vi "auto low bar and shoot.vi"(8 "high?":bool, 9 "Distance":dbl, 10 "defenseMode":dbl, 11 "RPM setting":dbl) -> ()   [LabVIEW 2015]
uses:
  <vilib>/Rock Robotics/WPI/Solenoid/WPI_SolenoidValue.ctl
  <vilib>/Rock Robotics/WPI/CAN/TalonSRX/WPI_CANTalonSRX_APIControlMode.ctl
  <vilib>/Rock Robotics/WPI/Solenoid/WPI_SolenoidSetEnum.vi
  <vilib>/Rock Robotics/Network Tables/NT Read Number.vi
  <vilib>/Rock Robotics/Network Tables/NT Read Boolean.vi
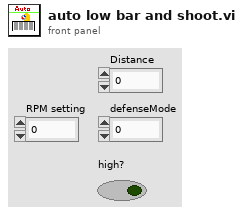
[diagram p1: front panel]
types:
  T1 = typedef "WPI_MotorControlDeviceRef.ctl" = cluster{"DeviceStatus":errorcluster, "Type":T2, "PWM":cluster{"PWM Channel":T3, "DeadBand":T4}, "CAN":cluster{"Device Number":u8, "Control Mode":T5, "Semaphore":T6, "Max Vout":dbl, "TalonSRX Control Mode":T7}, "Invert":bool}
  T2 = typedef "WPI_MotorControlType.ctl" = enum16{"PWM", "CAN", "CANTalonSRX"}
  T3 = typedef "FPGA_DIOPWMChannel.ctl" = enum8{"PWM 0", "PWM 1", "PWM 2", "PWM 3", "PWM 4", "PWM 5", "PWM 6", "PWM 7", "PWM 8", "PWM 9", "PWM MXP 0", "PWM MXP 1", "PWM MXP 2", "PWM MXP 3", "PWM MXP 4", "PWM MXP 5", "PWM MXP 6", "PWM MXP 7", "PWM MXP 8", "PWM MXP 9", "Invalid"}
  T4 = typedef "WPI_PWMDeadband.ctl" = cluster{"Name":string, "maxPositivePwm":i32, "minPositivePwm":i32, "centerPwm":i32, "maxNegativePwm":i32, "minNegativePwm":i32, "angularRange":u16}
  T5 = typedef "WPI_CANJaguar_ControlMode.ctl" = enum8{"Percent VBus", "Current", "Speed", "Position", "Voltage"}
  T6 = typedef "Semaphore RefNum" = refnum<k1>
  T7 = typedef "WPI_CANTalonSRX_APIControlMode.ctl" = enum8{"Percent VBus", "Speed", "Position", "Slave", "Unchanged / Invalid", "Voltage Compensation", "Current", "Motion Profile"}
  T8 = typedef "WPI_SolenoidDevRef.ctl" = cluster{"DevStatus":errorcluster, "Pneumatics Control Module":u8, "Forward Solenoid Channel":T9, "Reverse Solenoid Channel":T9}
  T9 = typedef "WPI_SolenoidChannel.ctl" = enum8{"Solenoid 0", "Solenoid 1", "Solenoid 2", "Solenoid 3", "Solenoid 4", "Solenoid 5", "Solenoid 6", "Solenoid 7", "Invalid"}
  T10 = typedef "WPI_GyroDevRef.ctl" = cluster{"DevStatus":errorcluster, "Analog Channel":T11, "Offset":dbl, "Gain (VoltsPerDegree/Second)":dbl, "Gyro Type":enum16{"Analog", "XRS450"}, "Handle":i32, "SPI Bus":T12, "Device Found":bool, "Sample Rate":dbl, "Calibrate On Open":bool}
  T11 = typedef "FPGA_AIChannel.ctl" = enum8{"AI 0", "AI 1", "AI 2", "AI 3", "AI MXP 0", "AI MXP 1", "AI MXP 2", "AI MXP 3", "Invalid"}
  T12 = typedef "spi_bus.ctl" = enum16{"SPI On-Board, CS0", "SPI On-Board, CS1", "SPI On-Board, CS2", "SPI On-Board, CS3", "SPI MXP", "Invalid"}
  T13 = typedef "WPI_SolenoidValue.ctl" = enum16{"Off", "On", "Forward", "Reverse"}
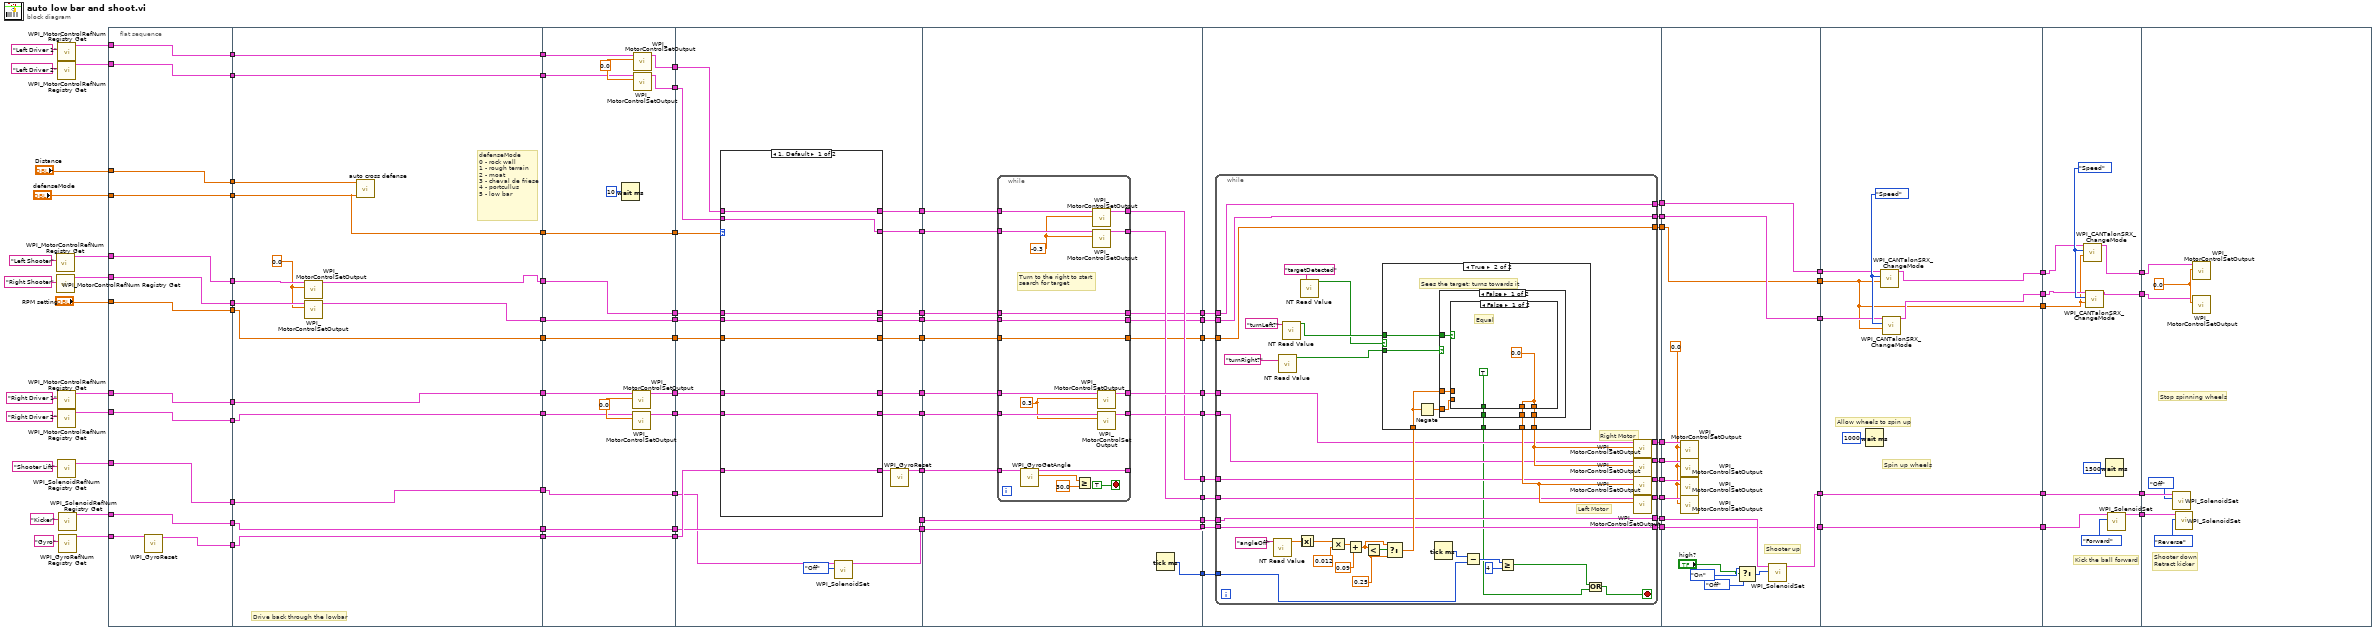
[diagram p0: block diagram]
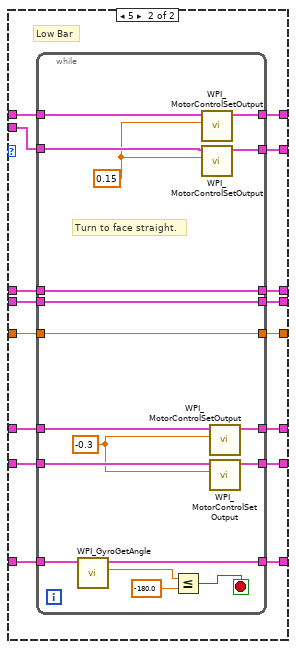
[diagram p2: hidden frame]
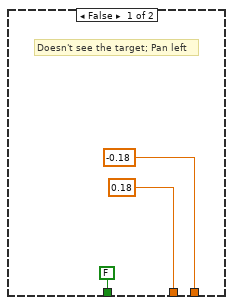
[diagram p3: hidden frame]
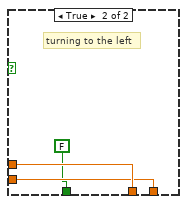
[diagram p4: hidden frame]
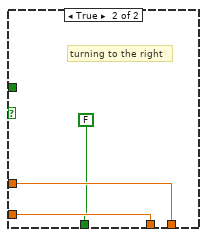
[diagram p5: hidden frame]
diagram:
  n1 = call <vilib>:"WPI_MotorControlRefNum Registry Get.vi"("refnum name"="Left Shooter") -> ("MotorControlDevRef"=w75:T1)  [unwired: 9 in, 1 out]
  n2 = call <vilib>:"WPI_MotorControlRefNum Registry Get.vi"("refnum name"="Right Shooter") -> ("MotorControlDevRef"=w72:T1)  [unwired: 9 in, 1 out]
  n3 = call <vilib>:"WPI_MotorControlRefNum Registry Get.vi"("refnum name"="Left Driver 1") -> ("MotorControlDevRef"=w98:T1)  [unwired: 9 in, 1 out]
  n4 = call <vilib>:"WPI_MotorControlRefNum Registry Get.vi"("refnum name"="Left Driver 2") -> ("MotorControlDevRef"=w97:T1)  [unwired: 9 in, 1 out]
  n5 = call <vilib>:"WPI_MotorControlRefNum Registry Get.vi"("refnum name"="Right Driver 1") -> ("MotorControlDevRef"=w96:T1)  [unwired: 9 in, 1 out]
  n6 = call <vilib>:"WPI_MotorControlRefNum Registry Get.vi"("refnum name"="Right Driver 2") -> ("MotorControlDevRef"=w95:T1)  [unwired: 9 in, 1 out]
  n7 = call <vilib>:"WPI_SolenoidRefNum Registry Get.vi"("refnum name"="Shooter Lift") -> ("SolenoidDevRef"=w90:T8)  [unwired: 9 in, 1 out]
  n8 = call <vilib>:"WPI_SolenoidRefNum Registry Get.vi"("refnum name"="Kicker") -> ("SolenoidDevRef"=w68:T8)  [unwired: 9 in, 1 out]
  n9 = call <vilib>:"WPI_GyroRefNum Registry Get.vi"("refnum name"="Gyro") -> ("GyroDevRef"=w86:T10)  [unwired: 9 in, 1 out]
  n10 = flat-sequence {
    tunnel: w95 -> [w108]
    tunnel: w96 -> [w109]
    tunnel: w97 -> [w110]
    tunnel: w98 -> [w111]
    tunnel: [w111] -> w94
    tunnel: [w110] -> w93
    tunnel: [w109] -> w92
    tunnel: [w108] -> w91
    tunnel: w90 -> [w99]
    tunnel: [w102] -> w87
    tunnel: w86 -> [w103]
    tunnel: [w107] -> w76
    tunnel: w75 -> [w107]
    tunnel: "RPM setting" -> [w106]
    tunnel: [w106] -> w73
    tunnel: w72 -> [w105]
    tunnel: [w105] -> w71
    tunnel: [w104] -> w69
    tunnel: w68 -> [w104]
    tunnel: [w99] -> w58
    tunnel: [w101] -> w57
    tunnel: "defenseMode" -> [w101]
    tunnel: "Distance" -> [w100]
    tunnel: [w100] -> w46
    tunnel: w94 -> [w126]
    tunnel: w93 -> [w125]
    tunnel: w92 -> [w122]
    tunnel: w91 -> [w121]
    tunnel: w87 -> [w119]
    tunnel: w76 -> [w116]
    tunnel: w73 -> [w124]
    tunnel: w71 -> [w115]
    tunnel: w69 -> [w118]
    tunnel: w58 -> [w120]
    tunnel: w57 -> [w117]
    tunnel: [w126] -> w55
    tunnel: [w125] -> w54
    tunnel: [w114] -> w52
    tunnel: [w113] -> w51
    tunnel: [w124] -> w49
    tunnel: w46 -> [w123]
    tunnel: [w122] -> w45
    tunnel: [w121] -> w44
    tunnel: [w120] -> w43
    tunnel: [w119] -> w41
    tunnel: [w118] -> w40
    tunnel: [w117] -> w36
    tunnel: [w142] -> w85
    tunnel: [w141] -> w84
    tunnel: [w140] -> w83
    tunnel: [w139] -> w82
    tunnel: [w128] -> w77
    tunnel: w55 -> [w137]
    tunnel: w54 -> [w136]
    tunnel: [w135] -> w53
    tunnel: w52 -> [w135]
    tunnel: w51 -> [w134]
    tunnel: [w134] -> w50
    tunnel: w49 -> [w133]
    tunnel: [w133] -> w48
    tunnel: w45 -> [w132]
    tunnel: w44 -> [w131]
    tunnel: w43 -> [w128]
    tunnel: [w130] -> w42
    tunnel: w41 -> [w130]
    tunnel: w40 -> [w129]
    tunnel: [w129] -> w39
    tunnel: [w127] -> w37
    tunnel: w36 -> [w127]
    tunnel: w85 -> [w163]
    tunnel: w84 -> [w162]
    tunnel: w83 -> [w165]
    tunnel: w82 -> [w164]
    tunnel: w77 -> [w153]
    tunnel: w53 -> [w152]
    tunnel: w50 -> [w150]
    tunnel: w48 -> [w148]
    tunnel: w42 -> [w161]
    tunnel: w39 -> [w154]
    tunnel: w37 -> [w166]
    tunnel: [w159] -> w35
    tunnel: [w158] -> w34
    tunnel: [w157] -> w33
    tunnel: [w156] -> w32
    tunnel: [w155] -> w31
    tunnel: [w154] -> w21
    tunnel: [w146] -> w19
    tunnel: [w151] -> w14
    tunnel: [w149] -> w13
    tunnel: [w147] -> w12
    tunnel: w35 -> [w226]
    tunnel: w34 -> [w225]
    tunnel: w33 -> [w224]
    tunnel: w32 -> [w223]
    tunnel: w31 -> [w222]
    tunnel: [w221] -> w30
    tunnel: [w220] -> w29
    tunnel: [w219] -> w28
    tunnel: [w218] -> w27
    tunnel: [w217] -> w22
    tunnel: w21 -> [w217]
    tunnel: w19 -> [w216]
    tunnel: [w216] -> w18
    tunnel: w14 -> [w215]
    tunnel: w13 -> [w214]
    tunnel: w12 -> [w213]
    tunnel: [w212] -> w10
    tunnel: [w211] -> w8
    tunnel: [w210] -> w6
    tunnel: [w209] -> w1
    tunnel: w30 -> [w263]
    tunnel: w29 -> [w262]
    tunnel: w28 -> [w261]
    tunnel: w27 -> [w260]
    tunnel: [w259] -> w26
    tunnel: [w258] -> w25
    tunnel: [w257] -> w24
    tunnel: [w256] -> w23
    tunnel: w22 -> [w255]
    tunnel: [w254] -> w20
    tunnel: w18 -> [w253]
    tunnel: [w252] -> w17
    tunnel: [w251] -> w11
    tunnel: w10 -> [w250]
    tunnel: [w249] -> w9
    tunnel: w8 -> [w248]
    tunnel: [w247] -> w7
    tunnel: w6 -> [w246]
    tunnel: w1 -> [w245]
    tunnel: [w336] -> w38
    tunnel: w26 -> [w335]
    tunnel: w25 -> [w334]
    tunnel: w24 -> [w333]
    tunnel: w23 -> [w332]
    tunnel: w20 -> [w329]
    tunnel: w17 -> [w330]
    tunnel: [w329] -> w15
    tunnel: w11 -> [w328]
    tunnel: w9 -> [w327]
    tunnel: w7 -> [w326]
    tunnel: [w328] -> w5
    tunnel: [w327] -> w4
    tunnel: [w326] -> w3
    tunnel: w38 -> [w348]
    tunnel: [w348] -> w66
    tunnel: [w347] -> w64
    tunnel: [w346] -> w62
    tunnel: [w344] -> w16
    tunnel: w15 -> [w344]
    tunnel: w5 -> [w343]
    tunnel: w4 -> [w342]
    tunnel: w3 -> [w341]
    tunnel: [w341] -> w2
    tunnel: [w358] -> w67
    tunnel: w66 -> [w358]
    tunnel: [w355] -> w65
    tunnel: w64 -> [w353]
    tunnel: [w354] -> w63
    tunnel: w62 -> [w352]
    tunnel: [w357] -> w61
    tunnel: w16 -> [w351]
    tunnel: w2 -> [w350]
    tunnel: w67 -> [w367]
    tunnel: w65 -> [w361]
    tunnel: w63 -> [w362]
    tunnel: w61 -> [w365]
    frame #0 {
      n11 = call <vilib>:"WPI_GyroReset.vi"("GyroDevRef"=w103) -> ("GyroDevRef"=w102:T10)  [unwired: 9 in, 1 out]
    }
    frame #1 {
      w112 = 0.0 ("Output")
      # "defenseMode\n0 - rock wall\n1 - rough terrain\n2 - moat\n3 - cheval de friese\n4 - portcullus\n5 - low bar"
      # "Drive back through the lowbar"
      n12 = call <vilib>:"WPI_MotorControlSetOutput.vi"("Output"=w112, "MotorControlDevRef"=w116) -> ("MotorControlDevRef"=w114:T1)  [unwired: 7 in, 2 out]
      n13 = call <vilib>:"WPI_MotorControlSetOutput.vi"("Output"=w112, "MotorControlDevRef"=w115) -> ("MotorControlDevRef"=w113:T1)  [unwired: 7 in, 2 out]
      n14 = call "auto cross defense.vi"("Defense type"=w117, "Distance"=w123) -> ()  [unwired: 10 in]
    }
    frame #2 {
      w143 = 0.0
      w144 = 0.0
      n15 = Wait (ms)(milliseconds to wait=u32 10) -> ()  [unwired: 1 out]
      n16 = call <vilib>:"WPI_MotorControlSetOutput.vi"("Output"=w143, "MotorControlDevRef"=w132) -> ("MotorControlDevRef"=w140:T1)  [unwired: 7 in, 2 out]
      n17 = call <vilib>:"WPI_MotorControlSetOutput.vi"("Output"=w143, "MotorControlDevRef"=w131) -> ("MotorControlDevRef"=w139:T1)  [unwired: 7 in, 2 out]
      n18 = call <vilib>:"WPI_MotorControlSetOutput.vi"("Output"=w144, "MotorControlDevRef"=w137) -> ("MotorControlDevRef"=w142:T1)  [unwired: 7 in, 2 out]
      n19 = call <vilib>:"WPI_MotorControlSetOutput.vi"("Output"=w144, "MotorControlDevRef"=w136) -> ("MotorControlDevRef"=w141:T1)  [unwired: 7 in, 2 out]
    }
    frame #3 {
      n20 = case shown="1, Default" w166 {
        tunnel: w165 -> [w171 w190]
        tunnel: w164 -> [w170 w189]
        tunnel: w163 -> [w173 w188]
        tunnel: w162 -> [w172 w187]
        tunnel: w161 -> [w174 w186]
        tunnel: [w174 w185] -> w160
        tunnel: [w171 w184] -> w158
        tunnel: [w170 w183] -> w157
        tunnel: [w173 w182] -> w156
        tunnel: [w172 w181] -> w155
        tunnel: w152 -> [w169 w180]
        tunnel: [w169 w179] -> w151
        tunnel: w150 -> [w168 w178]
        tunnel: [w168 w177] -> w149
        tunnel: [w167 w175] -> w147
        tunnel: w148 -> [w167 w176]
        frame 1, Default {
        }
        frame 5 {
          # "Low Bar"
          n21 = while {
            tunnel: w190 -> [w205]
            tunnel: w189 -> [w204]
            tunnel: w188 -> [w203]
            tunnel: w187 -> [w202]
            tunnel: w186 -> [w199]
            tunnel: [w198] -> w185
            tunnel: [w197] -> w184
            tunnel: [w196] -> w183
            tunnel: [w195] -> w182
            tunnel: [w194] -> w181
            tunnel: [w193] -> w179
            tunnel: w180 -> [w193]
            tunnel: [w192] -> w177
            tunnel: w178 -> [w192]
            tunnel: w176 -> [w191]
            tunnel: [w191] -> w175
            stop <- w208 stop-if-true
            w201 = -0.3 ("Output")
            w200 = 0.15
            # "Turn to face straight."
            n22 = call <vilib>:"WPI_GyroGetAngle.vi"("GyroDevRef"=w199) -> ("Angle"=w207:dbl, "GyroDevRef"=w198:T10)  [unwired: 6 in, 3 out]
            n23 = Less Or Equal?(x=w207, y=-180.0) -> (x <= y?=w208:bool)
            n24 = call <vilib>:"WPI_MotorControlSetOutput.vi"("Output"=w200, "MotorControlDevRef"=w203) -> ("MotorControlDevRef"=w195:T1)  [unwired: 7 in, 2 out]
            n25 = call <vilib>:"WPI_MotorControlSetOutput.vi"("Output"=w200, "MotorControlDevRef"=w202) -> ("MotorControlDevRef"=w194:T1)  [unwired: 7 in, 2 out]
            n26 = call <vilib>:"WPI_MotorControlSetOutput.vi"("Output"=w201, "MotorControlDevRef"=w205) -> ("MotorControlDevRef"=w197:T1)  [unwired: 7 in, 2 out]
            n27 = call <vilib>:"WPI_MotorControlSetOutput.vi"("Output"=w201, "MotorControlDevRef"=w204) -> ("MotorControlDevRef"=w196:T1)  [unwired: 7 in, 2 out]
          }
        }
      }
      n28 = call-poly <vilib>:"WPI_SolenoidSet.vi"("Value"=WPI_SolenoidValue."Off", "SolenoidDevRef"=w153) -> ("SolenoidDevRef"=w146:T8)  [unwired: 8 in, 1 out]
      n29 = call <vilib>:"WPI_GyroReset.vi"("GyroDevRef"=w160) -> ("GyroDevRef"=w159:T10)  [unwired: 9 in, 1 out]
    }
    frame #4 {
      n30 = while {
        tunnel: w225 -> [w242]
        tunnel: w224 -> [w241]
        tunnel: w223 -> [w240]
        tunnel: w222 -> [w239]
        tunnel: w226 -> [w236]
        tunnel: [w235] -> _
        tunnel: [w234] -> w221
        tunnel: [w233] -> w220
        tunnel: [w232] -> w219
        tunnel: [w231] -> w218
        tunnel: [w230] -> w212
        tunnel: w215 -> [w230]
        tunnel: [w229] -> w211
        tunnel: w214 -> [w229]
        tunnel: [w228] -> w210
        tunnel: w213 -> [w228]
        stop <- TRUE stop-if-true
        w238 = 0.3 ("Output")
        w237 = -0.3
        # "Turn to the right to start \nsearch for target"
        n31 = call <vilib>:"WPI_GyroGetAngle.vi"("GyroDevRef"=w236) -> ("Angle"=w244:dbl, "GyroDevRef"=w235:T10)  [unwired: 6 in, 3 out]
        n32 = Greater Or Equal?(x=w244, y=30.0) -> ()  [unwired: 1 out]
        n33 = call <vilib>:"WPI_MotorControlSetOutput.vi"("Output"=w237, "MotorControlDevRef"=w240) -> ("MotorControlDevRef"=w232:T1)  [unwired: 7 in, 2 out]
        n34 = call <vilib>:"WPI_MotorControlSetOutput.vi"("Output"=w237, "MotorControlDevRef"=w239) -> ("MotorControlDevRef"=w231:T1)  [unwired: 7 in, 2 out]
        n35 = call <vilib>:"WPI_MotorControlSetOutput.vi"("Output"=w238, "MotorControlDevRef"=w242) -> ("MotorControlDevRef"=w234:T1)  [unwired: 7 in, 2 out]
        n36 = call <vilib>:"WPI_MotorControlSetOutput.vi"("Output"=w238, "MotorControlDevRef"=w241) -> ("MotorControlDevRef"=w233:T1)  [unwired: 7 in, 2 out]
      }
      n37 = Tick Count (ms)() -> (millisecond timer value=w209:u32)
    }
    frame #5 {
      n38 = while {
        tunnel: w263 -> [w285]
        tunnel: w262 -> [w284]
        tunnel: w261 -> [w283]
        tunnel: w260 -> [w282]
        tunnel: [w279] -> w259
        tunnel: [w278] -> w258
        tunnel: [w277] -> w257
        tunnel: [w276] -> w256
        tunnel: [w275] -> w254
        tunnel: w255 -> [w275]
        tunnel: w253 -> [w274]
        tunnel: [w274] -> w252
        tunnel: [w273] -> w251
        tunnel: w250 -> [w273]
        tunnel: [w272] -> w249
        tunnel: w248 -> [w272]
        tunnel: [w271] -> w247
        tunnel: w246 -> [w271]
        tunnel: w245 -> [w269]
        stop <- w264 stop-if-true
        w288 = 0.25 ("y")
        # "Left Motor"
        # "Right Motor"
        n39 = call-poly <vilib>:"NT Read Value.vi"("Name"="angleOff") -> ("Numeric"=w298:dbl)  [unwired: 9 in, 1 out]
        n40 = call-poly <vilib>:"NT Read Value.vi"("Name"="turnRight?") -> ("Boolean"=w297:bool)  [unwired: 9 in, 1 out]
        n41 = call-poly <vilib>:"NT Read Value.vi"("Name"="turnLeft?") -> ("Boolean"=w296:bool)  [unwired: 9 in, 1 out]
        n42 = Absolute Value(x=w298) -> (abs(x)=w293:dbl)
        n43 = call-poly <vilib>:"NT Read Value.vi"("Name"="targetDetected") -> ("Boolean"=w280:bool)  [unwired: 9 in, 1 out]
        n44 = Multiply(x=w293, y=0.012) -> (x*y=w291:dbl)
        n45 = Add(x=w291, y=0.09) -> (x+y=w287:dbl)
        n46 = Less?(x=w287, y=w288) -> (x < y?=w289:bool)
        n47 = Select(t=w287, s=w289, f=w288) -> (s? t:f=w286:dbl)
        n48 = case shown="True" w280 {
          tunnel: [-0.18 w311] -> w301
          tunnel: [0.18 w310] -> w300
          tunnel: w297 -> [_ w308]
          tunnel: w296 -> [_ w307]
          tunnel: w286 -> [_ w306]
          tunnel: [FALSE w305] -> w266
          frame False {
            # "Doesn't see the target; Pan left"
          }
          frame True {
            # "Sees the target; turns towards it"
            n49 = Negate(x=w306) -> (-x=w309:dbl)
            n50 = case shown="False" w308 {
              tunnel: w306 -> [w316 w325]
              tunnel: [w315 w325] -> w311
              tunnel: [w317 w324] -> w310
              tunnel: w309 -> [w314 w324]
              tunnel: w307 -> [w313 _]
              tunnel: [w312 FALSE] -> w305
              frame False {
                n51 = case shown="False" w313 {
                  tunnel: [w319 w322] -> w317
                  tunnel: w316 -> [_ w322]
                  tunnel: [w319 w321] -> w315
                  tunnel: w314 -> [_ w321]
                  tunnel: [TRUE FALSE] -> w312
                  frame False {
                    w319 = 0.0
                    # "Equal"
                  }
                  frame True {
                    # "turning to the left"
                  }
                }
              }
              frame True {
                # "turning to the right"
              }
            }
          }
        }
        n52 = Tick Count (ms)() -> (millisecond timer value=w270:u32)
        n53 = Subtract(x=w270, y=w269) -> (x-y=w268:u32)
        n54 = Greater Or Equal?(x=w268, y=u32 4) -> (x >= y?=w265:bool)
        n55 = Or(x=w265, y=w266) -> (x .or. y?=w264:bool)
        n56 = call <vilib>:"WPI_MotorControlSetOutput.vi"("Output"=w301, "MotorControlDevRef"=w285) -> ("MotorControlDevRef"=w279:T1)  [unwired: 7 in, 2 out]
        n57 = call <vilib>:"WPI_MotorControlSetOutput.vi"("Output"=w301, "MotorControlDevRef"=w284) -> ("MotorControlDevRef"=w278:T1)  [unwired: 7 in, 2 out]
        n58 = call <vilib>:"WPI_MotorControlSetOutput.vi"("Output"=w300, "MotorControlDevRef"=w283) -> ("MotorControlDevRef"=w277:T1)  [unwired: 7 in, 2 out]
        n59 = call <vilib>:"WPI_MotorControlSetOutput.vi"("Output"=w300, "MotorControlDevRef"=w282) -> ("MotorControlDevRef"=w276:T1)  [unwired: 7 in, 2 out]
      }
    }
    frame #6 {
      w331 = 0.0
      # "Shooter up"
      n60 = call <vilib>:"WPI_MotorControlSetOutput.vi"("Output"=w331, "MotorControlDevRef"=w335) -> ()  [unwired: 7 in, 3 out]
      n61 = call <vilib>:"WPI_MotorControlSetOutput.vi"("Output"=w331, "MotorControlDevRef"=w334) -> ()  [unwired: 7 in, 3 out]
      n62 = call <vilib>:"WPI_MotorControlSetOutput.vi"("Output"=w331, "MotorControlDevRef"=w333) -> ()  [unwired: 7 in, 3 out]
      n63 = call <vilib>:"WPI_MotorControlSetOutput.vi"("Output"=w331, "MotorControlDevRef"=w332) -> ()  [unwired: 7 in, 3 out]
      n64 = Select(t=WPI_SolenoidValue."On" ("Value"), s="high?", f=WPI_SolenoidValue."Off") -> (s? t:f=w340:T13)
      n65 = call-poly <vilib>:"WPI_SolenoidSet.vi"("Value"=w340, "SolenoidDevRef"=w330) -> ("SolenoidDevRef"=w336:T8)  [unwired: 8 in, 1 out]
    }
    frame #7 {
      w345 = WPI_CANTalonSRX_APIControlMode."Speed" ("Control Mode")
      # "Allow wheels to spin up"
      # "Spin up wheels"
      n66 = Wait (ms)(milliseconds to wait=u32 1000) -> ()  [unwired: 1 out]
      n67 = call <vilib>:"WPI_CANTalonSRX_ChangeMode.vi"("Output"=w341, "Control Mode"=w345, "CAN Talon SRX Ref"=w343) -> ("CAN Talon SRX Ref"=w347:T1)  [unwired: 7 in, 1 out]
      n68 = call <vilib>:"WPI_CANTalonSRX_ChangeMode.vi"("Output"=w341, "Control Mode"=w345, "CAN Talon SRX Ref"=w342) -> ("CAN Talon SRX Ref"=w346:T1)  [unwired: 7 in, 1 out]
    }
    frame #8 {
      w356 = WPI_CANTalonSRX_APIControlMode."Speed" ("Control Mode")
      # "Kick the ball forward"
      n69 = call <vilib>:"WPI_CANTalonSRX_ChangeMode.vi"("Output"=w350, "Control Mode"=w356, "CAN Talon SRX Ref"=w353) -> ("CAN Talon SRX Ref"=w355:T1)  [unwired: 7 in, 1 out]
      n70 = call <vilib>:"WPI_CANTalonSRX_ChangeMode.vi"("Output"=w350, "Control Mode"=w356, "CAN Talon SRX Ref"=w352) -> ("CAN Talon SRX Ref"=w354:T1)  [unwired: 7 in, 1 out]
      n71 = Wait (ms)(milliseconds to wait=u32 1500) -> ()  [unwired: 1 out]
      n72 = call-poly <vilib>:"WPI_SolenoidSet.vi"("Value"=WPI_SolenoidValue."Forward", "SolenoidDevRef"=w351) -> ("SolenoidDevRef"=w357:T8)  [unwired: 8 in, 1 out]
    }
    frame #9 {
      w363 = 0.0
      # "Stop spinning wheels"
      # "Shooter down\nRetract kicker"
      n73 = call-poly <vilib>:"WPI_SolenoidSet.vi"("Value"=WPI_SolenoidValue."Off", "SolenoidDevRef"=w367) -> ()  [unwired: 8 in, 2 out]
      n74 = call-poly <vilib>:"WPI_SolenoidSet.vi"("Value"=WPI_SolenoidValue."Reverse", "SolenoidDevRef"=w365) -> ()  [unwired: 8 in, 2 out]
      n75 = call <vilib>:"WPI_MotorControlSetOutput.vi"("Output"=w363, "MotorControlDevRef"=w361) -> ()  [unwired: 7 in, 3 out]
      n76 = call <vilib>:"WPI_MotorControlSetOutput.vi"("Output"=w363, "MotorControlDevRef"=w362) -> ()  [unwired: 7 in, 3 out]
    }
  }
